vi "Fibonacci_Sequence_Solution.vi"(4 "Sequence Size":i32) -> (1 "Fibonacci Sequence":i32[](array[numeric]))   [LabVIEW 2013]
panel:
  # "Fibonacci Sequence\n\nCreate a VI that takes one numeric input which specifies the number of Fibonacci numbers to\n generate returns an array containing the specified number of numbers of Fibonacci sequence."
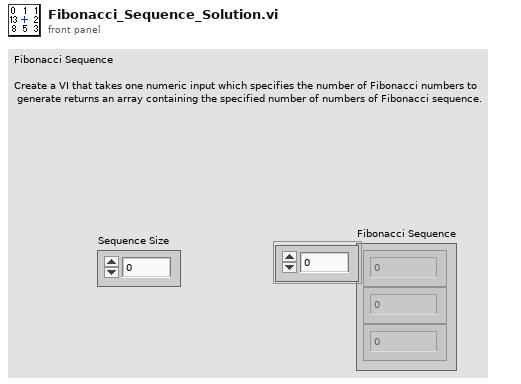
[diagram p1: front panel]
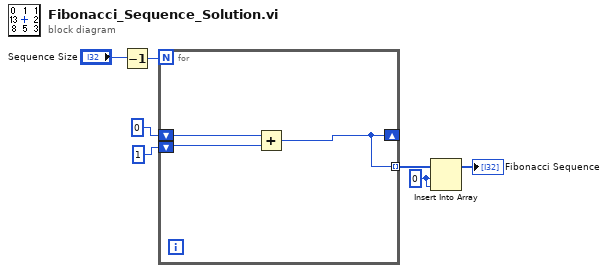
[diagram p0: block diagram]
diagram:
  w2 = 0 ("index")
  n1 = Decrement(x="Sequence Size") -> (x-1=w4:i32)
  n2 = for {
    N: w4 -> [_]
    shift-right: [w8] -> _
    shift-left: 0 ("Sequence Size") -> [w10]
    shift-left: 1 ("Sequence Size") -> [w9]
    tunnel: [w8] -> w3 mode=indexing
    n3 = Add(x=w10, y=w9) -> (x+y=w8:i32)
  }
  n4 = Insert Into Array(array=w3, index=w2, new element=w2) -> (→"Fibonacci Sequence":i32[])
